vi "Get Relay Names.vi"(8 "error in (no error)":errorcluster, 11 "Route Manager in":refnum<class "Route Manager.lvclass">) -> (0 "error out":errorcluster, 2 "relay strings":string[](array[string]), 3 "Route Manager out":refnum<class "Route Manager.lvclass">)   [LabVIEW 2015, in "Route Manager.lvclass"]
uses:
  Route Manager.lvclass
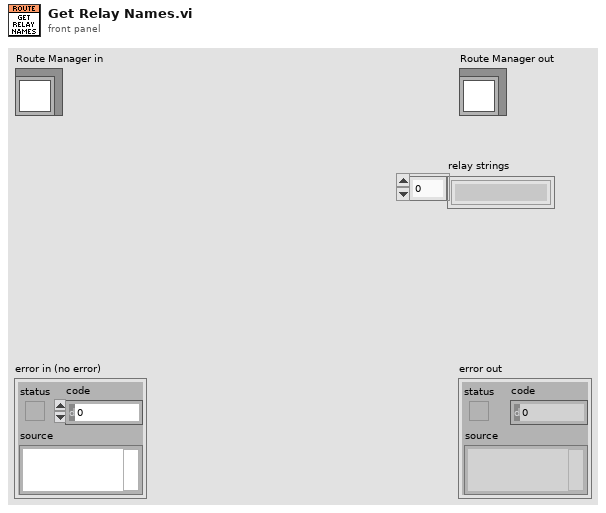
[diagram p1: front panel]
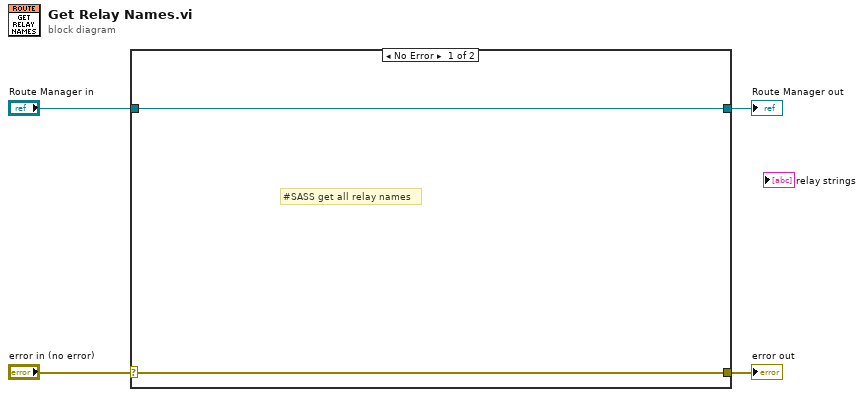
[diagram p0: block diagram]
diagram:
  n1 = case shown="No Error" "error in (no error)" {
    selector: "error in (no error)" -> [w6 w8]
    tunnel: [w6 w8] -> w3
    tunnel: [w5 w7] -> w1
    tunnel: "Route Manager in" -> [w5 w7]
    frame No Error {
      # "#SASS get all relay names"
    }
    frame Error {
    }
  }
  "error out" <- w3
  "Route Manager out" <- w1
